vi "Destructor.vi"(8 "error in (no error)":errorcluster, 11 "Vapour Generator in":refnum<class "Vapour Generator.lvclass">) -> (0 "error out":errorcluster, 3 "Vapour Generator out":refnum<class "Vapour Generator.lvclass">)   [LabVIEW 2011, in "Vapour Generator.lvclass"]
uses:
  Vapour Generator.lvclass
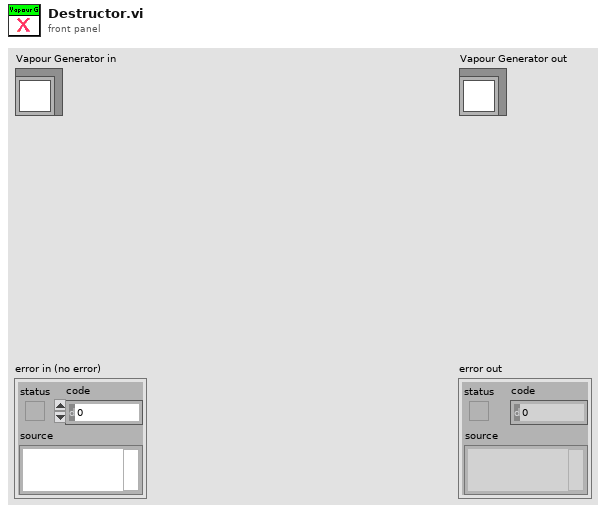
[diagram p1: front panel]
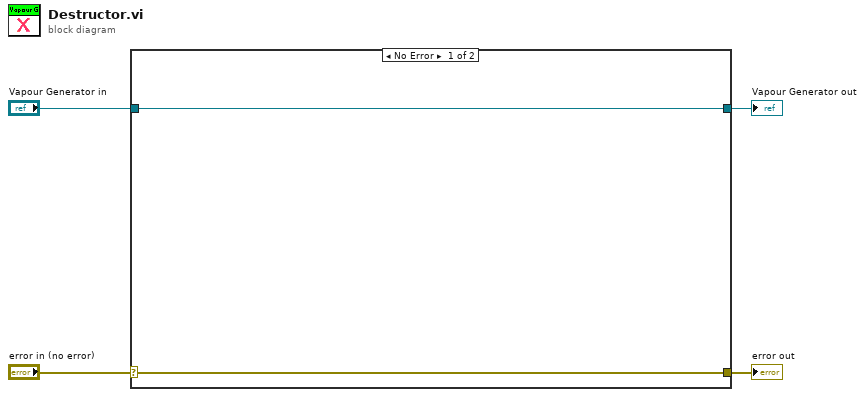
[diagram p0: block diagram]
diagram:
  n1 = case shown="No Error" "error in (no error)" {
    selector: "error in (no error)" -> [w5 w8]
    tunnel: [w5 w8] -> w3
    tunnel: [w6 w7] -> w1
    tunnel: "Vapour Generator in" -> [w6 w7]
    frame No Error {
    }
    frame Error {
    }
  }
  "error out" <- w3
  "Vapour Generator out" <- w1
